vi "Check Uesr found.vi"(8 "error in (no error)":errorcluster, 9 "Password":string, 10 "Username":string, 11 "Credential info":string[][](array[string])) -> (0 "error out":errorcluster, 2 "Index":i32, 3 "Found?":bool)   [LabVIEW 2016, in "User Interface.lvlib"]
uses:
  User Interface.lvlib
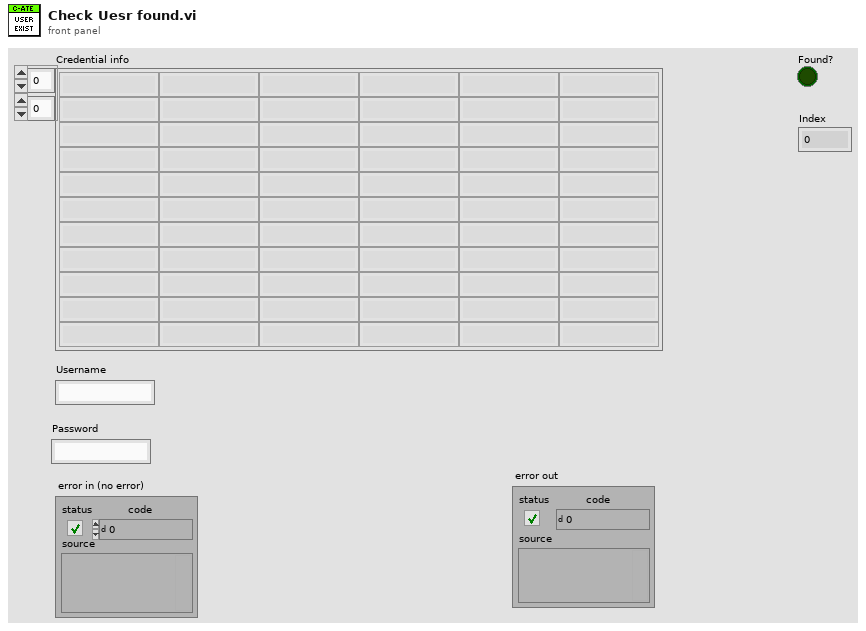
[diagram p1: front panel]
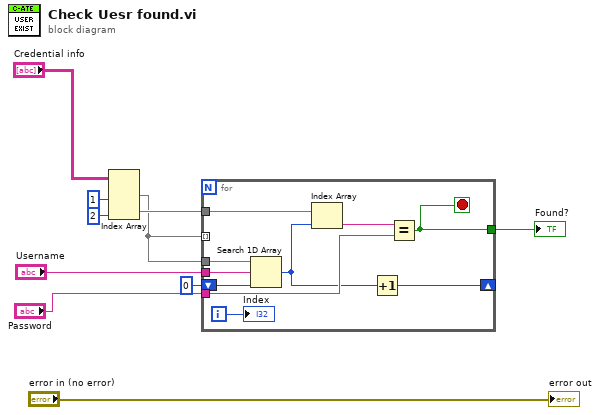
[diagram p0: block diagram]
diagram:
  n1 = Index Array(array="Credential info", index (col) #1=1 ("disabled index (col)"), index (col) #2=2 ("index (col)")) -> (element #1=w6:string[], element #2=w8:string[])  [unwired: 2 in]
  n2 = for {
    tunnel: "Username" -> [w20]
    tunnel: w6 -> [w15]
    tunnel: w8 -> [w19]
    tunnel: "Password" -> [w17]
    tunnel: [w16] -> w7
    tunnel: w6 -> [_] mode=indexing
    shift-right: [w12] -> _
    shift-left: 0 -> [w13]
    i -> [w11]
    stop <- w16 stop-if-true
    n3 = Search 1D Array(1D array=w15, element=w20, start index (0)=w13) -> (index of element=w14:i32)
    n4 = Index Array(array=w19, index=w14) -> (element=w18:string)
    n5 = Increment(x=w14) -> (x+1=w12:i32)
    n6 = Equal?(x=w18, y=w17) -> (x = y?=w16:bool)
    "Index" <- w11
  }
  "Found?" <- w7
  "error out" <- "error in (no error)"
